vi "MTS_InterpolPower.vi"(1 "Desired Power ( µW )":dbl, 2 "Positions":dbl[](array[numeric]), 3 "Intensitys":dbl[](array[numeric])) -> (0 "Numeric":dbl)   [LabVIEW 2011]
uses:
  <vilib>/gmath/NI_Gmath.lvlib
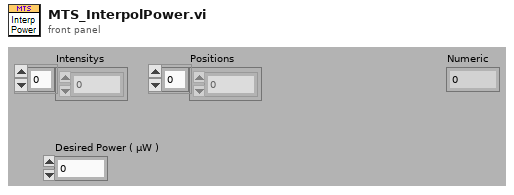
[diagram p1: front panel]
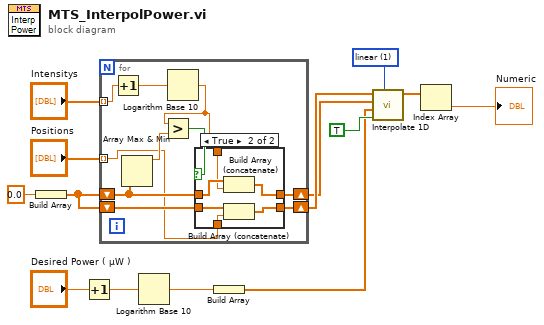
[diagram p0: block diagram]
diagram:
  w11 = 1 items=["nearest", "linear", "spline", "cubic Hermite", "Lagrange"] ("method")
  n1 = Build Array(0.0 ("Desired Power ( µW )")) -> (w7:dbl[])
  n2 = Increment(x="Desired Power ( µW )") -> (x+1=w2:dbl)
  n3 = for {
    tunnel: "Intensitys" -> [w16] mode=indexing
    tunnel: "Positions" -> [w18] mode=indexing
    shift-right: [w21] -> w4
    shift-left: w7 -> [w22]
    shift-right: [w20] -> w5
    shift-left: w7 -> [w19]
    n4 = Increment(x=w16) -> (x+1=w17:dbl)
    n5 = Array Max & Min(array=w22) -> (max value=w24:dbl)  [unwired: 3 out]
    n6 = Logarithm Base 10(1:w17) -> (0:w15:dbl)
    n7 = Greater?(x=w15, y=w24) -> (0:w23:bool)
    n8 = case shown="True" w23 {
      tunnel: w22 -> [w26 w32]
      tunnel: [w26 w31] -> w21
      tunnel: [w25 w29] -> w20
      tunnel: w19 -> [w25 w30]
      tunnel: w15 -> [_ w28]
      tunnel: w18 -> [_ w27]
      frame False {
      }
      frame True {
        n9 = Build Array (concatenate)(w32, w28) -> (w31:dbl[])
        n10 = Build Array (concatenate)(w30, w27) -> (w29:dbl[])
      }
    }
  }
  n11 = Logarithm Base 10(1:w2) -> (0:w1:dbl)
  n12 = Build Array(w1) -> (w6:dbl[])
  n13 = call <vilib>:"Interpolate 1D.vi"("method"=w11, "X is monotonic"=TRUE, "xi"=w6, "X"=w4, "Y"=w5) -> ("yi"=w12:dbl[])  [unwired: 4 in, 2 out]
  n14 = Index Array(array=w12) -> (element=→"Numeric":dbl)  [unwired: 1 in]
